vi "Core_[HSMS]Selected_Send Message_Retry.vi"(8 "error in (no error)":errorcluster, 9 "SECS-II Class":refnum<class "SECS-II Class.lvclass">, 10 "Reply Notifier":refnum<notifier>, 11 "HSMS Class in":refnum<class "HSMS Class.lvclass">) -> (0 "error out":errorcluster, 3 "HSMS Class out":refnum<class "HSMS Class.lvclass">)   [LabVIEW 2020, in "SECS Communication.lvlib" / "HSMS Class.lvclass"]
uses:
  HSMS Class.lvclass
  SECS-II Class/SECS-II Class.lvclass
  HSMS Class.lvclass/HSMS Class.ctl
  Notifier Type.ctl
  HSMS State.ctl
  Read T3(Reply Timeout).vi
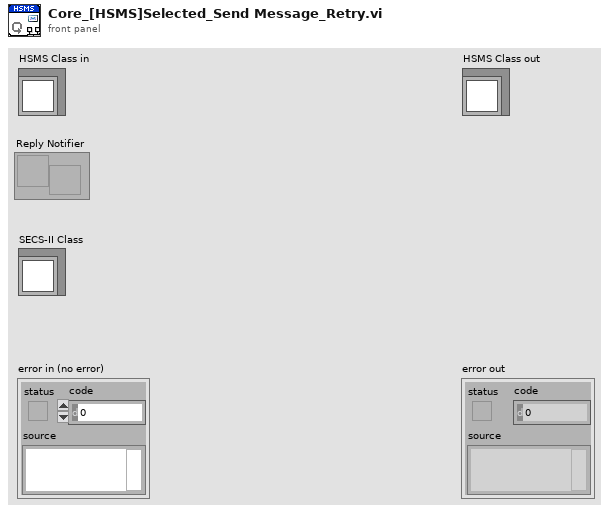
[diagram p1: front panel]
types:
  T1 = typedef "SECS Communication.lvlib/HSMS Class.lvclass/Notifier Type.ctl" = enum16{"TCPIP Connect", "TCPIP Disconnect", "Receive Message", "Send Message", "T3 Timeout", "T6 Timeout", "T7 Timeout", "Error", "Stop"}
  T2 = typedef "SECS Communication.lvlib/HSMS Class.lvclass/HSMS State.ctl" = enum16{"[TCP/IP]Not Connect", "[HSMS]Not Selected", "[HSMS]Selected", "Stop"}
  T3 = typedef "SECS Communication.lvlib/HSMS Class.lvclass/Message Packet.ctl" = cluster{"Message Header Cluster":T4, "Message Header":u8[], "Message Text":u8[]}
  T4 = typedef "SECS Communication.lvlib/HSMS Class.lvclass/Message Header.ctl" = cluster{"Byte 0-1(Session ID)":u16, "W-Bit":bool, "Byte 2":u8, "Byte 3":u8, "Byte 4(PType)":T5, "Byte 5(SType)":T6, "Byte 6-9(System Btyes)":u8[]}
  T5 = typedef "SECS Communication.lvlib/HSMS Class.lvclass/PType.ctl" = enum8{"SECS-II Encoding", "Reserved"}
  T6 = typedef "SECS Communication.lvlib/HSMS Class.lvclass/SType.ctl" = enum8{"Data Message", "Select.req", "Select.rsp", "Deselect.req", "Deselect.rsp", "Linktest.req", "Linktest.rsp", "Reject.req", "Separate.req"}
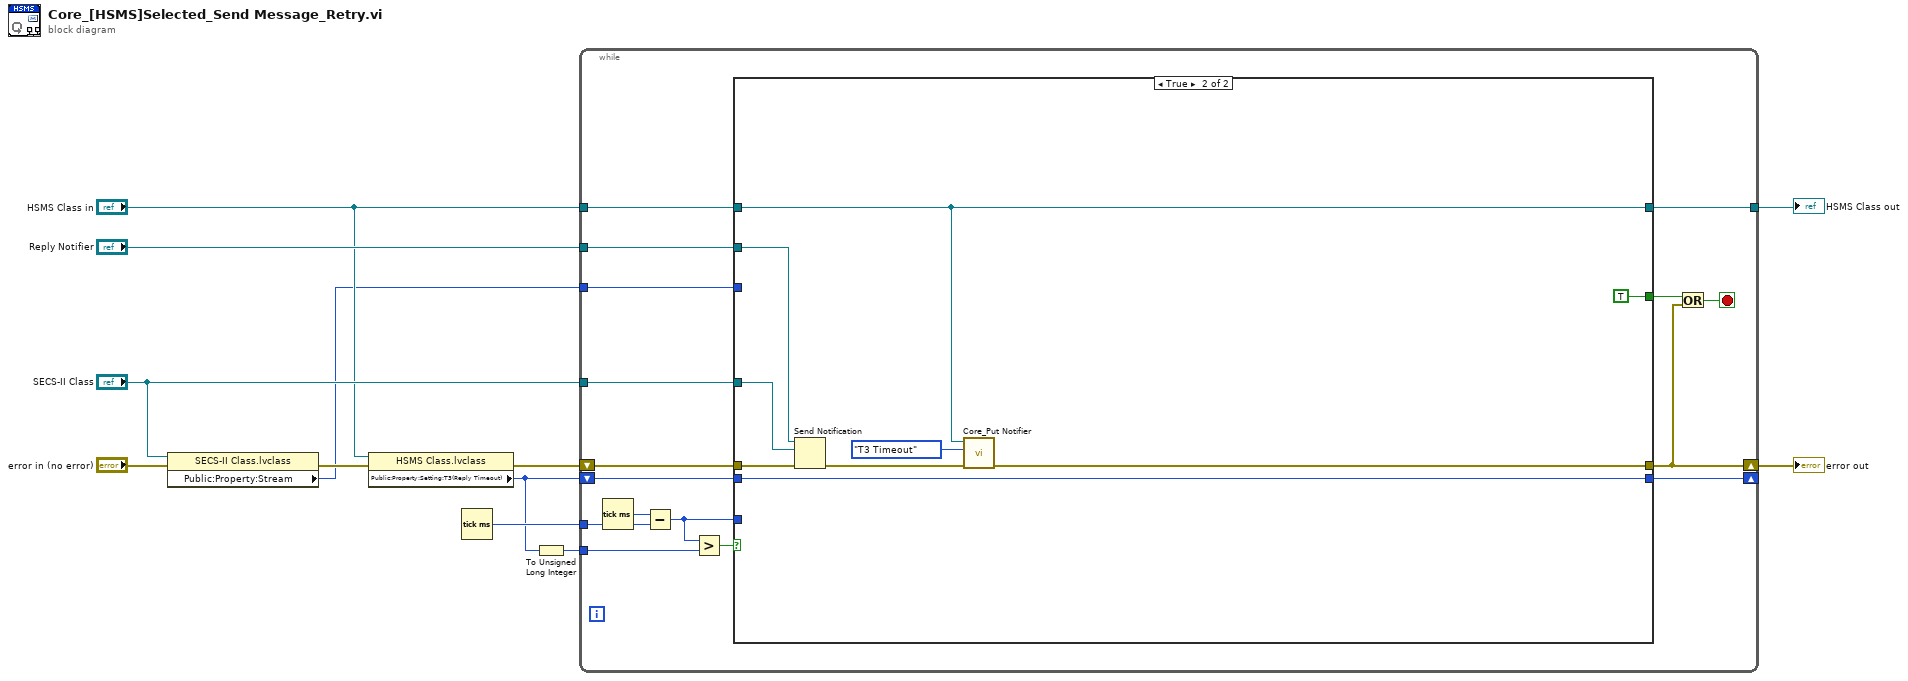
[diagram p0: block diagram]
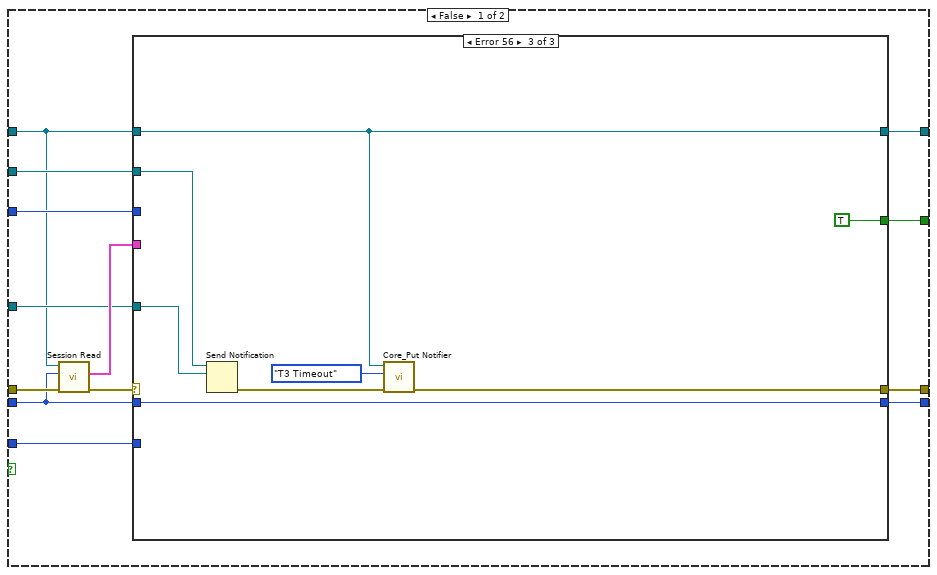
[diagram p2: hidden frame]
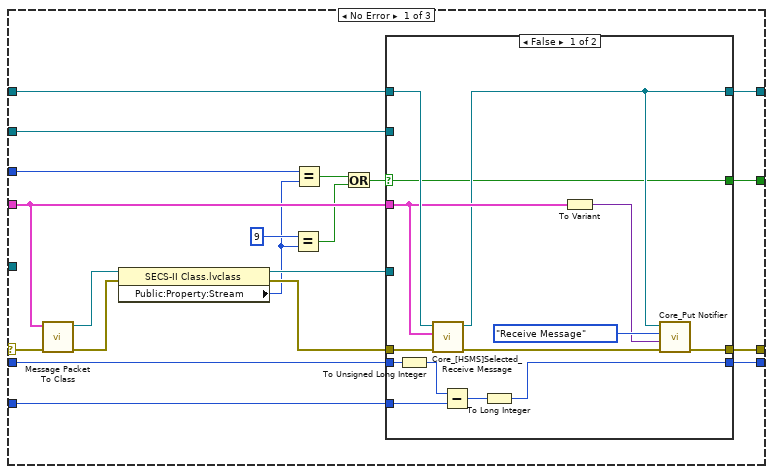
[diagram p3: hidden frame]
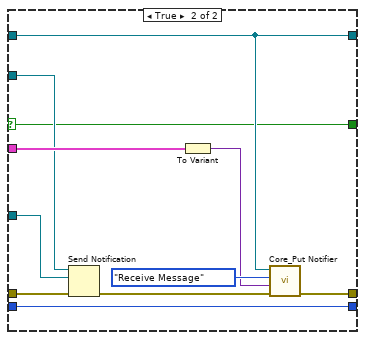
[diagram p4: hidden frame]
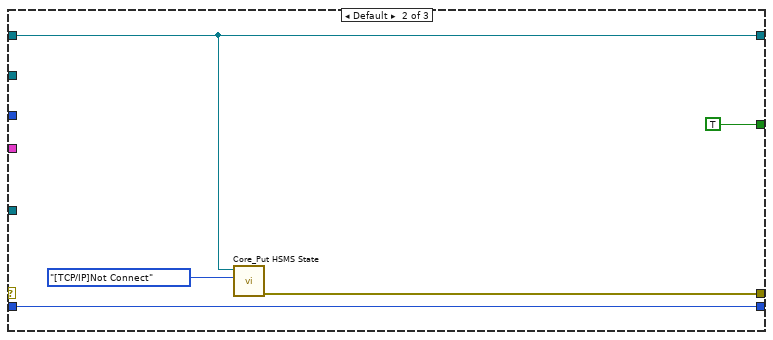
[diagram p5: hidden frame]
diagram:
  n1 = property class="SECS-II Class.lvclass"(reference="SECS-II Class", error in="error in (no error)") -> (error out=w2:errorcluster, "Public:Property:Stream"=w1:u8)  [unwired: 1 out]
  n2 = property class="HSMS Class.lvclass"(reference="HSMS Class in", error in=w2) -> (error out=w6:errorcluster, "Public:Property:Setting:T3(Reply Timeout)"=w3:i32)  [unwired: 1 out]
  n3 = Tick Count (ms)() -> (millisecond timer value=w5:u32)
  n4 = To Unsigned Long Integer(number=w3) -> (unsigned 32bit integer=w4:u32)
  n5 = while {
    tunnel: "Reply Notifier" -> [w27]
    tunnel: "SECS-II Class" -> [w26]
    tunnel: w1 -> [w25]
    shift-right: [w14] -> w12
    shift-left: w6 -> [w23]
    tunnel: "HSMS Class in" -> [w24]
    tunnel: [w28] -> w11
    tunnel: w5 -> [w21]
    tunnel: w4 -> [w20]
    shift-right: [w16] -> _
    shift-left: w3 -> [w22]
    stop <- w13 stop-if-true
    n6 = Tick Count (ms)() -> (millisecond timer value=w18:u32)
    n7 = Subtract(x=w18, y=w21) -> (x-y=w17:u32)
    n8 = Greater?(x=w17, y=w20) -> (0:w19:bool)
    n9 = case shown="True" w19 {
      tunnel: [w40 w102] -> w14
      tunnel: [w39 w103] -> w28
      tunnel: w27 -> [w38 w105]
      tunnel: w26 -> [w37 w104]
      tunnel: w25 -> [w35 _]
      tunnel: w24 -> [w34 w103]
      tunnel: w23 -> [w33 w106]
      tunnel: w22 -> [w30 w100]
      tunnel: [w32 TRUE] -> w15
      tunnel: w17 -> [w31 _]
      tunnel: [w29 w100] -> w16
      frame False {
        n10 = call "Session Read.vi"("error in (no error)"=w33, "Timeout"=w30, "HSMS Class in"=w34) -> ("error out"=w36:errorcluster, "Message Packet"=w41:T3)  [unwired: 6 in, 1 out]
        n11 = case shown="Error 56" w36 {
          selector: w36 -> [w61 _ _]
          tunnel: [w59 w89 w98] -> w40
          tunnel: w41 -> [w58 _ _]
          tunnel: w34 -> [w60 w90 w97]
          tunnel: [w55 w90 w97] -> w39
          tunnel: w37 -> [_ _ w95]
          tunnel: w38 -> [w57 _ w94]
          tunnel: w35 -> [w56 _ _]
          tunnel: [w54 TRUE TRUE] -> w32
          tunnel: w31 -> [w53 _ _]
          tunnel: w30 -> [w52 w87 w92]
          tunnel: [w51 w87 w92] -> w29
          frame No Error {
            n12 = call "Message Packet To Class.vi"("error in"=w61, "Message Packet"=w58) -> ("error out"=w44:errorcluster, "SECS-II Class"=w43:refnum<class "SECS-II Class.lvclass">)  [unwired: 7 in, 1 out]
            n13 = property class="SECS-II Class.lvclass"(reference=w43, error in=w44) -> (reference out=w49:refnum<class "SECS-II Class.lvclass">, error out=w50:errorcluster, "Public:Property:Stream"=w42:u8)
            n14 = Equal?(x=u8 9, y=w42) -> (x = y?=w46:bool)
            n15 = Equal?(x=w56, y=w42) -> (x = y?=w47:bool)
            n16 = Or(x=w47, y=w46) -> (x .or. y?=w45:bool)
            n17 = case shown="False" w45 {
              selector: w45 -> [w67 w78]
              tunnel: w60 -> [w74 w79]
              tunnel: [w68 w84] -> w59
              tunnel: w58 -> [w70 w83]
              tunnel: w57 -> [_ w81]
              tunnel: w50 -> [w75 w80]
              tunnel: [w69 w79] -> w55
              tunnel: [w67 w78] -> w54
              tunnel: w53 -> [w66 _]
              tunnel: w52 -> [w65 w77]
              tunnel: [w62 w77] -> w51
              tunnel: w49 -> [_ w76]
              frame False {
                n18 = To Unsigned Long Integer(number=w65) -> (unsigned 32bit integer=w64:u32)
                n19 = call "Core_[HSMS]Selected_Receive Message.vi"("error in (no error)"=w75, "Message Packet"=w70, "HSMS Class in"=w74) -> ("error out"=w71:errorcluster, "HSMS Class out"=w69:refnum<class "HSMS Class.lvclass">)  [unwired: 7 in]
                n20 = Subtract(x=w64, y=w66) -> (x-y=w63:u32)
                n21 = To Long Integer(number=w63) -> (32bit integer=w62:i32)
                n22 = To Variant(anything=w70) -> (Variant=w72:variant)
                n23 = call "Core_Put Notifier.vi"("error in (no error)"=w71, "Data"=w72, "Notifier Type"=Notifier_Type."Receive Message", "HSMS Class in"=w69) -> ("error out"=w68:errorcluster)  [unwired: 6 in, 1 out]
              }
              frame True {
                n24 = Send Notification(notification=w76, notifier=w81, error in (no error)=w80) -> (error out=w85:errorcluster)  [unwired: 1 out]
                n25 = To Variant(anything=w83) -> (Variant=w82:variant)
                n26 = call "Core_Put Notifier.vi"("error in (no error)"=w85, "Data"=w82, "Notifier Type"=Notifier_Type."Receive Message", "HSMS Class in"=w79) -> ("error out"=w84:errorcluster)  [unwired: 6 in, 1 out]
              }
            }
          }
          frame Default {
            n27 = call "Core_Put HSMS State.vi"("HSMS State"=HSMS_State."[TCP/IP]Not Connect", "HSMS Class in"=w90) -> ("error out"=w89:errorcluster)  [unwired: 8 in, 1 out]
          }
          frame Error {
            n28 = Send Notification(notification=w95, notifier=w94) -> (error out=w96:errorcluster)  [unwired: 1 in, 1 out]
            n29 = call "Core_Put Notifier.vi"("error in (no error)"=w96, "Notifier Type"=Notifier_Type."T3 Timeout", "HSMS Class in"=w97) -> ("error out"=w98:errorcluster)  [unwired: 7 in, 1 out]
          }
        }
      }
      frame True {
        n30 = Send Notification(notification=w104, notifier=w105, error in (no error)=w106) -> (error out=w107:errorcluster)  [unwired: 1 out]
        n31 = call "Core_Put Notifier.vi"("error in (no error)"=w107, "Notifier Type"=Notifier_Type."T3 Timeout", "HSMS Class in"=w103) -> ("error out"=w102:errorcluster)  [unwired: 7 in, 1 out]
      }
    }
    n32 = Or(x=w15, y=w14) -> (x .or. y?=w13:bool)
  }
  "error out" <- w12
  "HSMS Class out" <- w11
